vi "Clear Hardware.vi"(2 "error in (no error)":errorcluster, 3 "Aerotech_Soloist in":refnum<class "Aerotech_Soloist.lvclass">) -> (0 "error out":errorcluster, 1 "Aerotech_Soloist out":refnum<class "Aerotech_Soloist.lvclass">)   [LabVIEW 2013, in "Aerotech_Soloist.lvclass"]
doc: "This VI resets any necessary hardware so that the device will be ready for the next run."
uses:
  Aerotech_Soloist.lvclass
  Device/Device.lvclass
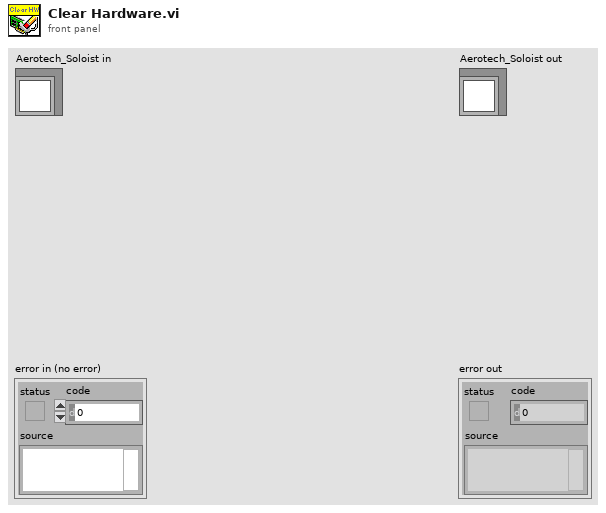
[diagram p1: front panel]
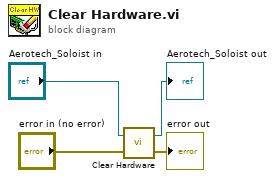
[diagram p0: block diagram]
diagram:
  n1 = call-parent "Clear Hardware.vi"("error in (no error)"="error in (no error)", "Device in"="Aerotech_Soloist in") -> ("error out"=→"error out":errorcluster, "Device out"=→"Aerotech_Soloist out":refnum<class "Aerotech_Soloist.lvclass">)
